vi "Emballage_Bdd_Affiche_ChoixListe.vi"(8 "entrée d'erreur (pas d'erreur)":errorcluster, 10 "Tableau_indice":i32[](array[numeric]), 11 "tableau des produits code FAS":string[](array[string])) -> (0 "sortie d'erreur":errorcluster, 3 "Produit_code_FAS":string)   [LabVIEW 2020]
panel:
  in  "Bouton OK":bool
  in  "Liste déroulante":i32(listbox)
  # "Plusieurs produits correspondent au code barre scanné.\nVeuillez sélectionner le produit correspondant!!"
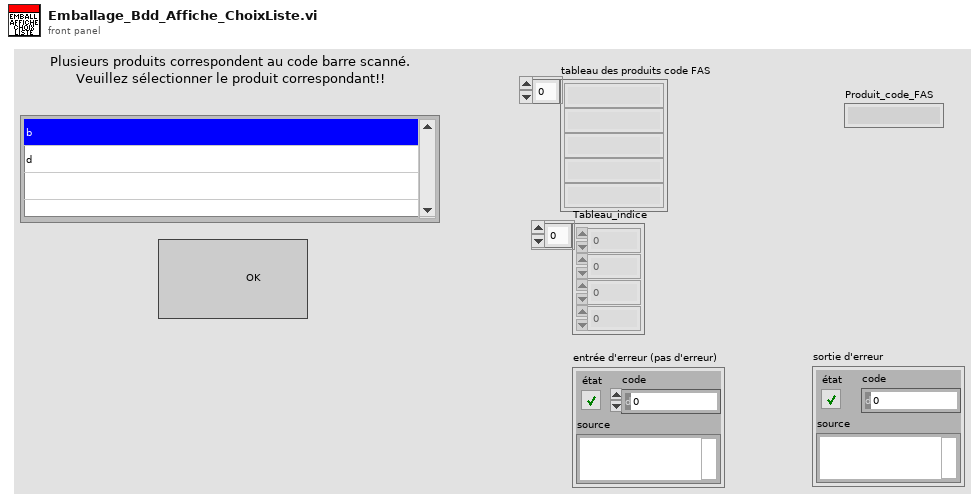
[diagram p1: front panel]
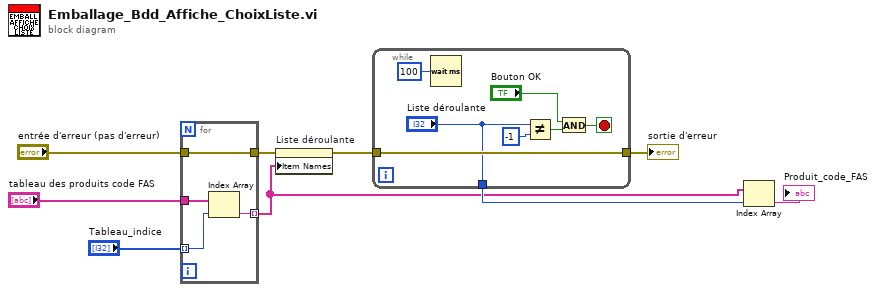
[diagram p0: block diagram]
diagram:
  n1 = for {
    tunnel: "Tableau_indice" -> [w12] mode=indexing
    tunnel: "tableau des produits code FAS" -> [w13]
    tunnel: [w11] -> w2 mode=indexing
    tunnel: [w10] -> w8
    tunnel: "entrée d'erreur (pas d'erreur)" -> [w10]
    n2 = Index Array(array=w13, index=w12) -> (element=w11:string)
  }
  n3 = property on="Liste déroulante" class="LstDér (strict)"(error in=w8, "Item Names"=w2) -> (error out=w6:errorcluster)  [unwired: 1 in, 1 out]
  n4 = while {
    tunnel: w6 -> [w16]
    tunnel: [w16] -> w5
    tunnel: ["Liste déroulante"] -> w3
    stop <- w19 stop-if-true
    n5 = Wait (ms)(milliseconds to wait=u32 100 ("attente (ms)")) -> ()  [unwired: 1 out]
    n6 = Not Equal?(x="Liste déroulante", y=-1) -> (x != y?=w18:bool)
    n7 = And(x="Bouton OK", y=w18) -> (x .and. y?=w19:bool)
  }
  "sortie d'erreur" <- w5
  n8 = Index Array(array=w2, index=w3) -> (element=→"Produit_code_FAS":string)
